vi "Lab 9 Exercise 1.vi"() -> ()   [LabVIEW 2023]
panel:
  out "XY Graph":cluster{i32[], dbl[]}(graph)
  out "pi/2?":dbl
  in  "# Needles":i32
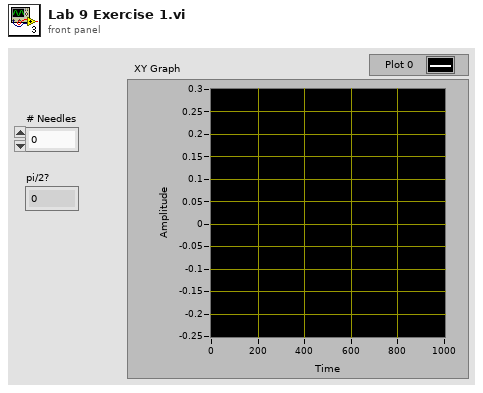
[diagram p1: front panel]
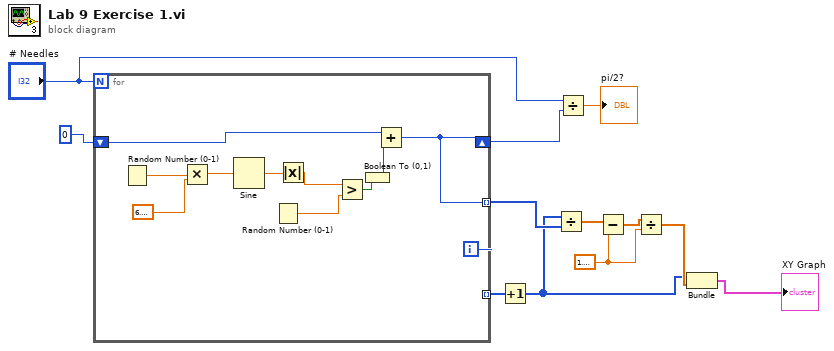
[diagram p0: block diagram]
diagram:
  w5 = 1.5707963267948966
  n1 = for {
    N: "# Needles" -> [_]
    shift-right: [w14] -> w10
    shift-left: 0 -> [w21]
    tunnel: [w14] -> w8 mode=indexing
    tunnel: [w13] -> w4 mode=indexing
    i -> [w13]
    n2 = Random Number (0-1)() -> (number: 0 to 1=w23:dbl)
    n3 = Multiply(x=w23, y=6.283185307179586) -> (x*y=w20:dbl)
    n4 = Sine(x=w20) -> (sin(x)=w19:dbl)
    n5 = Random Number (0-1)() -> (number: 0 to 1=w17:dbl)
    n6 = Absolute Value(x=w19) -> (abs(x)=w18:dbl)
    n7 = Greater?(x=w18, y=w17) -> (0:w16:bool)
    n8 = Boolean To (0,1)(Boolean=w16) -> (0, 1=w15:i16)
    n9 = Add(x=w21, y=w15) -> (x+y=w14:i32)
  }
  n10 = Increment(x=w4) -> (x+1=w1:i32[])
  n11 = Divide(x=w1, y=w8) -> (x/y=w7:dbl[])
  n12 = Divide(x="# Needles", y=w10) -> (x/y=→"pi/2?":dbl)
  n13 = Subtract(x=w7, y=w5) -> (x-y=w6:dbl[])
  n14 = Divide(x=w6, y=w5) -> (x/y=w3:dbl[])
  n15 = Bundle(w1, w3) -> (→"XY Graph":cluster{i32[], dbl[]})  [unwired: 1 in]
